vi "Class to Variant.vi"(8 "error in (no error)":errorcluster, 10 "Data in":variant, 11 "LabVIEW Build Node in":refnum<class "LabVIEW Build Node.lvclass">) -> (0 "error out":errorcluster, 1 "Serialized Object Name":string, 2 "Data":variant, 3 "LabVIEW Build Node out":refnum<class "LabVIEW Build Node.lvclass">)   [LabVIEW 2014, in "LabVIEW Build Node.lvclass"]
uses:
  LabVIEW Build Node.lvclass
  Shared/Controls/LabVIEW Build - STYP.ctl
  LabVIEW Build Node.lvclass/LabVIEW Build Node.ctl
  Classes/Build Job/Build Job.lvclass
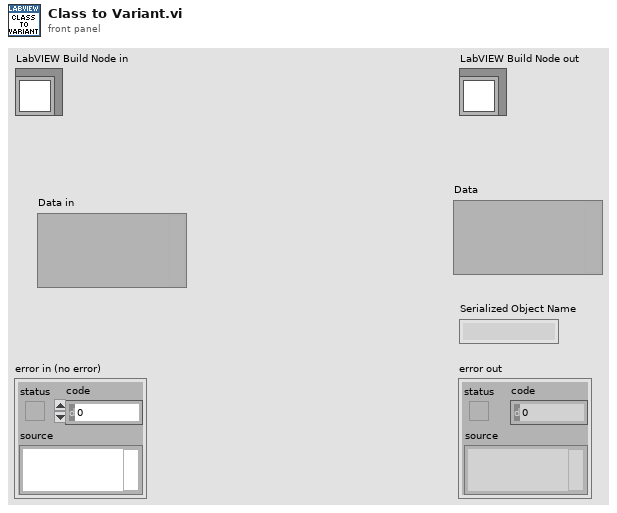
[diagram p1: front panel]
types:
  T1 = typedef "LabVIEW Build - STYP.ctl" = cluster{"Executor_Number":string, "Workspace_Path":string, "Build_Spec":string, "Target":string, "Project_Path":string, "Auto_Version_Increment":bool}
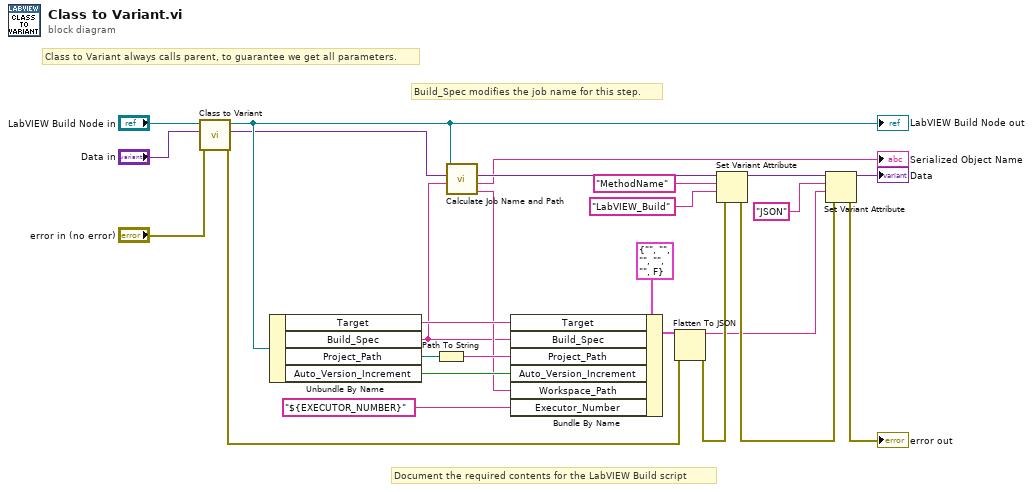
[diagram p0: block diagram]
diagram:
  # "Document the required contents for the LabVIEW Build script"
  # "Build_Spec modifies the job name for this step."
  # "Class to Variant always calls parent, to guarantee we get all parameters."
  n1 = call-parent "Class to Variant.vi"("error in (no error)"="error in (no error)", "Data in"="Data in", "Build Job in"="LabVIEW Build Node in") -> ("error out"=w18:errorcluster, "Data Out"=w9:variant, "Build Job out"=w12:refnum<class "LabVIEW Build Node.lvclass">)  [unwired: 5 in, 1 out]
  "LabVIEW Build Node out" <- w12
  n2 = Unbundle By Name(w12) -> ("Target"=w5:string, "Build_Spec"=w1:string, "Project_Path"=w14:path, "Auto_Version_Increment"=w13:bool)
  n3 = Path To String(path=w14) -> (string=w10:string)
  n4 = call "Calculate Job Name and Path.vi"("Job Target"=w1, "Data in"=w9, "Build Job"=w12) -> ("Workspace Path"=w3:string, "Job Name"=→"Serialized Object Name":string, "Data out"=w4:variant)  [unwired: 6 in]
  n5 = Bundle By Name(cluster=T1 {"Executor_Number"="", "Workspace_Path"="", "Build_Spec"="", "Target"="", "Project_Path"="", "Auto_Version_Increment"=FALSE} ("LabVIEW Build"), "Target"=w5, "Build_Spec"=w1, "Project_Path"=w10, "Auto_Version_Increment"=w13, "Workspace_Path"=w3, "Executor_Number"="${EXECUTOR_NUMBER}") -> (w24:T1)
  n6 = Flatten To JSON(anything=w24, error in (no error)=w18) -> (JSON string=w6:string, 11:w11:errorcluster)  [unwired: 1 in]
  n7 = Set Variant Attribute(Variant=w4, name="MethodName", value="LabVIEW_Build", error in=w11) -> (Variant out=w17:variant, error out=w16:errorcluster)  [unwired: 1 out]
  n8 = Set Variant Attribute(Variant=w17, name="JSON" ("Name"), value=w6, error in=w16) -> (Variant out=→"Data":variant, error out=→"error out":errorcluster)  [unwired: 1 out]
